vi "Periodic Tasks.vi"(8 "error in":errorcluster) -> ()   [LabVIEW 2019]
doc: "This VI runs in parallel to other tasks. It can contain as many user-defined periodic loops as you need. These can carry out PID or other sorts of timed response."
uses:
  <vilib>/Rock Robotics/WPI/Solenoid/WPI_SolenoidValue.ctl
  <vilib>/Rock Robotics/WPI/Utilities/WPI_GetSetVariantRefNum.vi
  <vilib>/Rock Robotics/Network Tables/NT Write Boolean.vi
  <vilib>/Rock Robotics/WPI/Solenoid/WPI_SolenoidSetEnum.vi
panel:
  in  "Output 3":dbl=-0.8 format="%#_13g"
  in  "Bottom":dbl=-1.0 format="%#_13g"
  in  "Top":dbl=0.27 format="%#_13g"
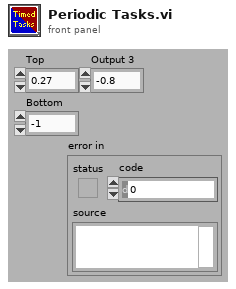
[diagram p1: front panel]
types:
  T1 = typedef "WPI_JoystickDevRef.ctl" = cluster{"Device":T2}
  T2 = typedef "WPI_JoystickDeviceEnum.ctl" = enum16{"USB 0", "USB 1", "USB 2", "USB 3", "USB 4", "USB 5"}
  T3 = typedef "WPI_SolenoidValue.ctl" = enum16{"Off", "On", "Forward", "Reverse"}
  T4 = typedef "WPI_SolenoidDevRef.ctl" = cluster{"DevStatus":errorcluster, "Pneumatics Control Module":u8, "Forward Solenoid Channel":T5, "Reverse Solenoid Channel":T5}
  T5 = typedef "WPI_SolenoidChannel.ctl" = enum8{"Solenoid 0", "Solenoid 1", "Solenoid 2", "Solenoid 3", "Solenoid 4", "Solenoid 5", "Solenoid 6", "Solenoid 7", "Invalid"}
  T6 = typedef "WPI_MotorControlDeviceRef.ctl" = cluster{"DeviceStatus":errorcluster, "Type":T7, "PWM":cluster{"PWM Channel":T8, "DeadBand":T9}, "CAN":cluster{"Device Number":u8, "SetOutput VI Ref":variant, "GetOutput VI Ref":variant, "Enable VI Ref":variant, "Disable VI Ref":variant, "Data":variant}, "Invert":bool, "DIO PWM":cluster{"PWM \"Enable\" Channel":T8, "DIOChannel":T10, "PWM Rate":dbl}}
  T7 = typedef "WPI_MotorControlType.ctl" = enum16{"PWM", "CAN", "DIO PWM"}
  T8 = typedef "FPGA_DIOPWMChannel.ctl" = enum8{"PWM 0", "PWM 1", "PWM 2", "PWM 3", "PWM 4", "PWM 5", "PWM 6", "PWM 7", "PWM 8", "PWM 9", "PWM MXP 0", "PWM MXP 1", "PWM MXP 2", "PWM MXP 3", "PWM MXP 4", "PWM MXP 5", "PWM MXP 6", "PWM MXP 7", "PWM MXP 8", "PWM MXP 9", "Invalid"}
  T9 = typedef "WPI_PWMDeadband.ctl" = cluster{"Name":string, "maxPositivePwm":i32, "minPositivePwm":i32, "centerPwm":i32, "maxNegativePwm":i32, "minNegativePwm":i32, "angularRange":u16}
  T10 = typedef "FPGA_DIOChannel.ctl" = enum8{"DIO 0", "DIO 1", "DIO 2", "DIO 3", "DIO 4", "DIO 5", "DIO 6", "DIO 7", "DIO 8", "DIO 9", "DIO MXP 0", "DIO MXP 1", "DIO MXP 2", "DIO MXP 3", "DIO MXP 4", "DIO MXP 5", "DIO MXP 6", "DIO MXP 7", "DIO MXP 8", "DIO MXP 9", "DIO MXP 10", "DIO MXP 11", "DIO MXP 12", "DIO MXP 13", "DIO MXP 14", "DIO MXP 15", "SPI Port CS1", "SPI Port CS2", "SPI Port CS3", "SPI Port MISO", "SPI Port MOSI", "Invalid"}
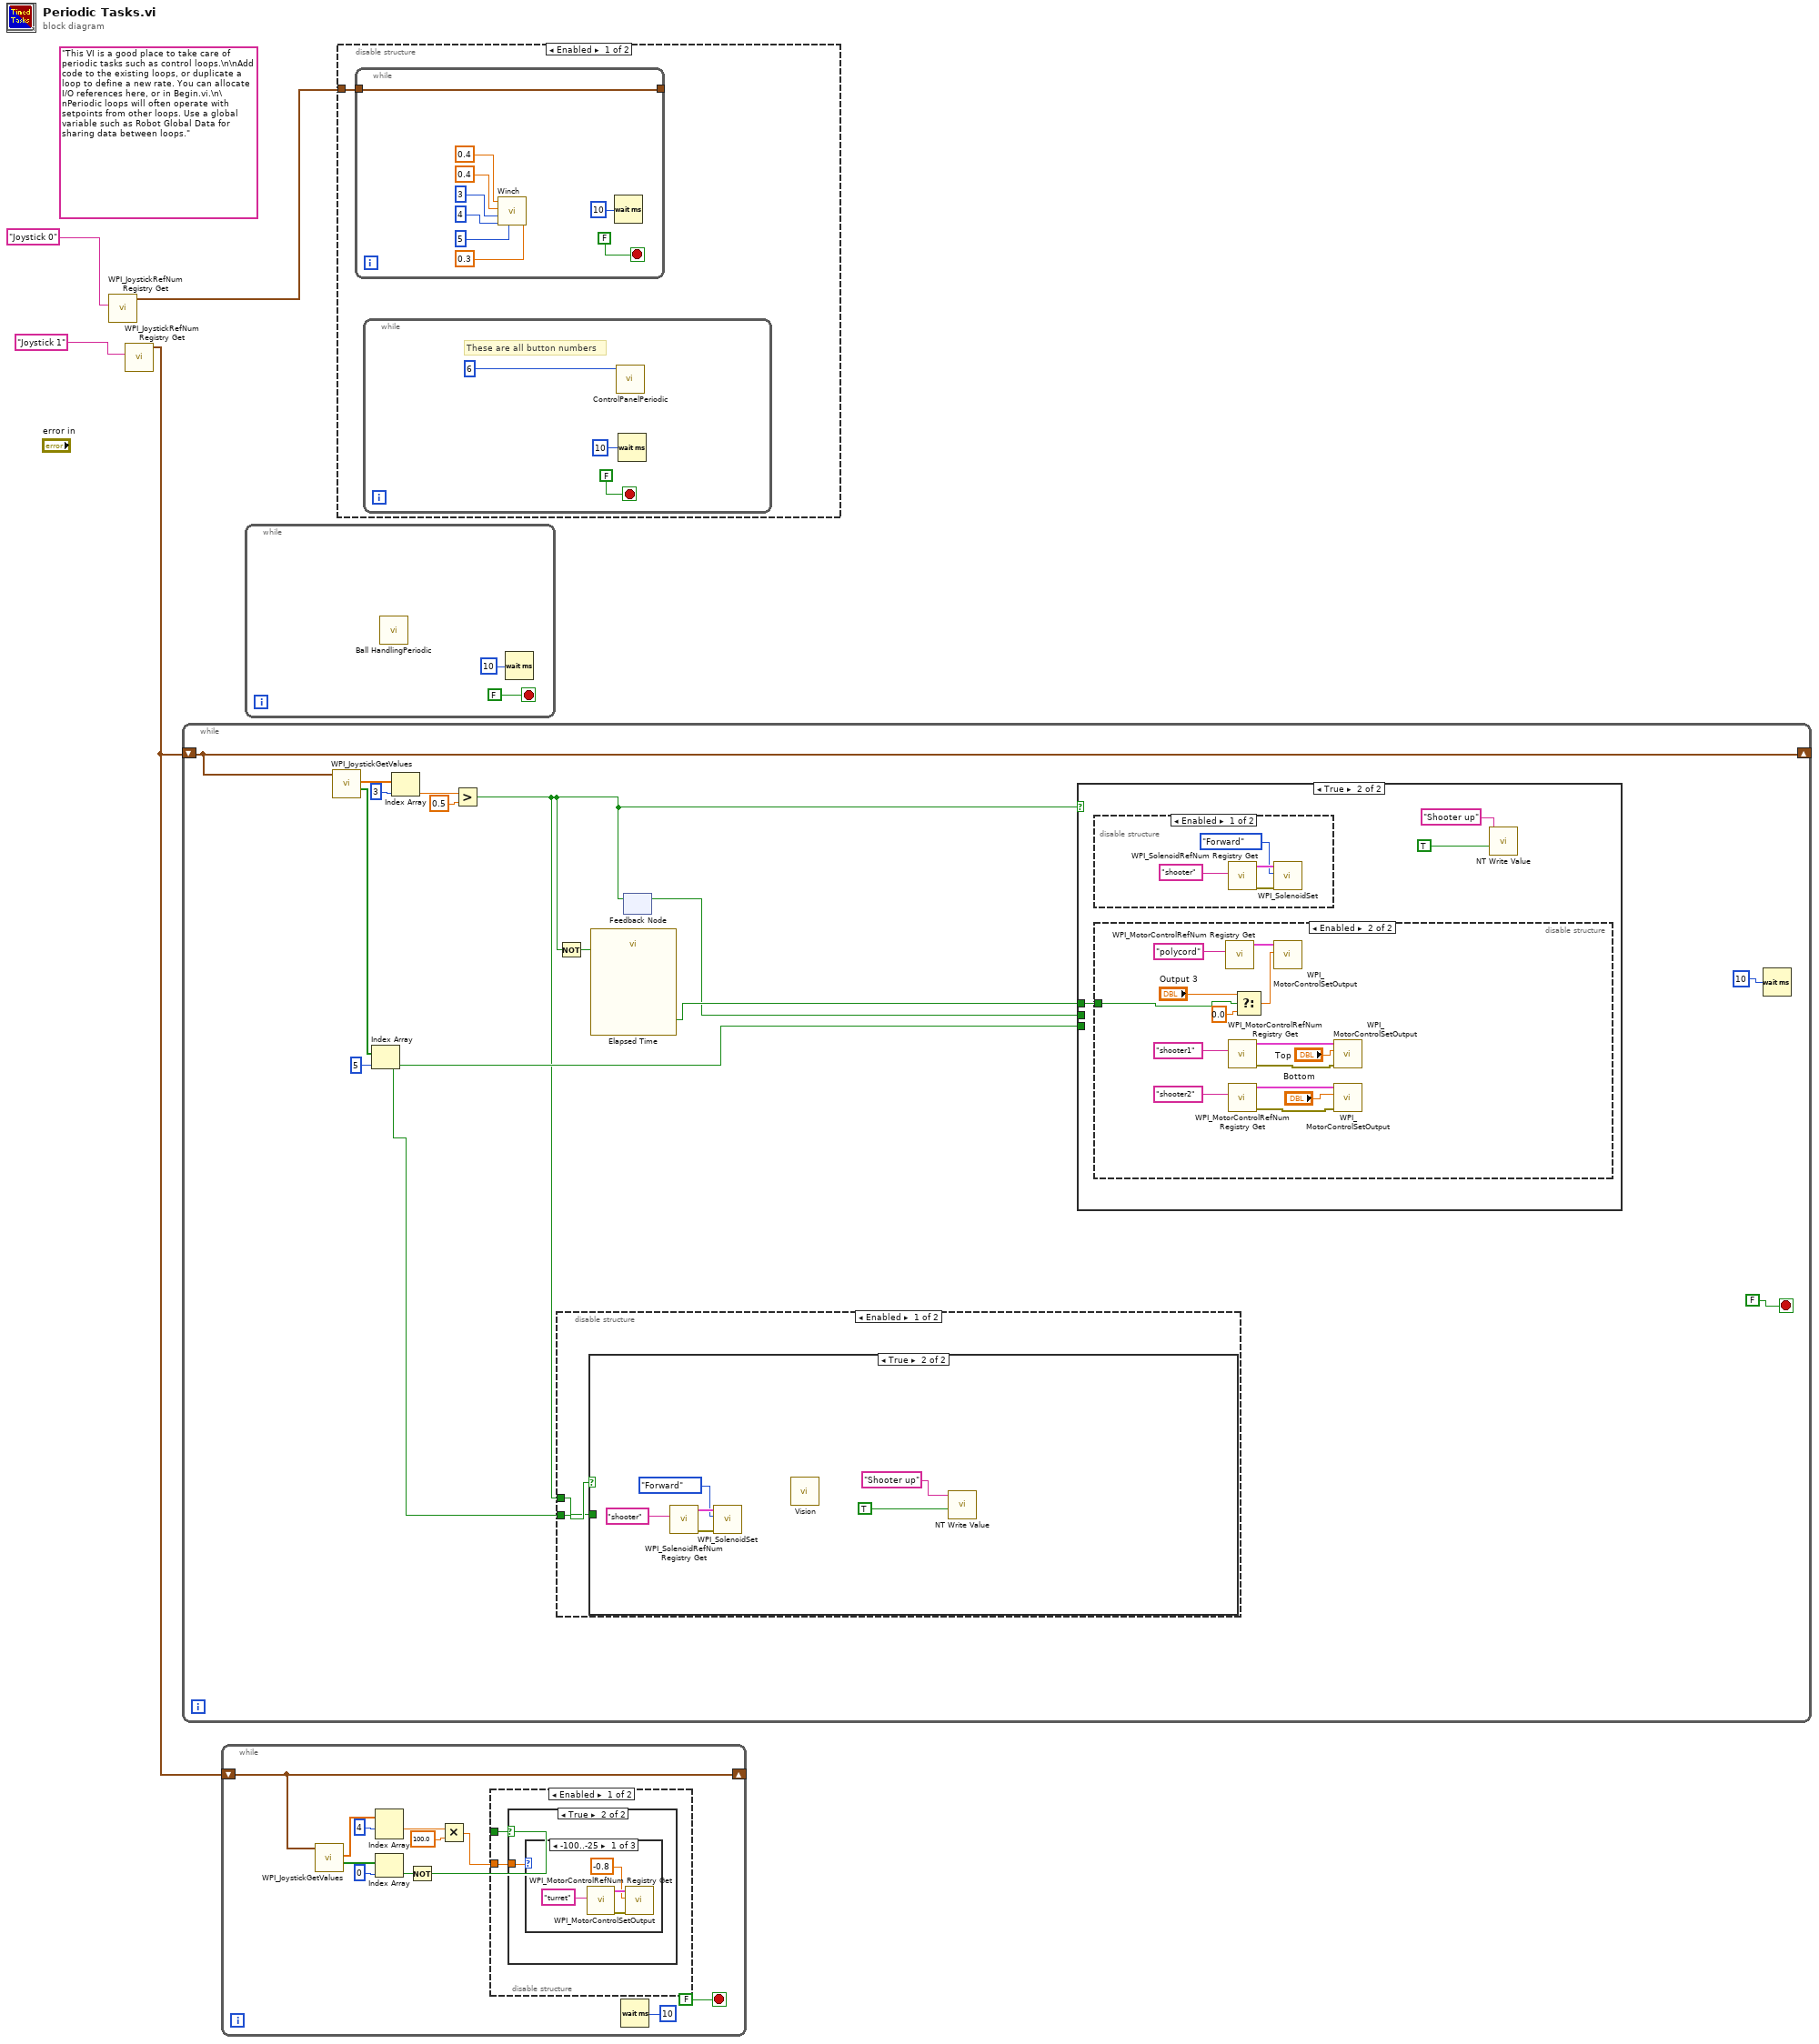
[diagram p0: block diagram]
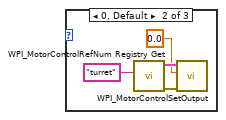
[diagram p3: hidden frame]
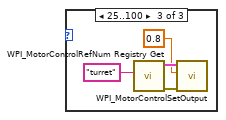
[diagram p4: hidden frame]
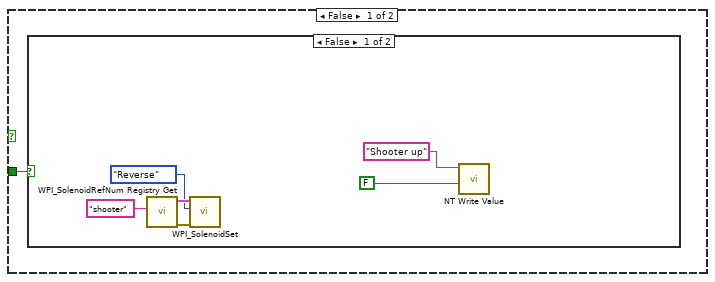
[diagram p6: hidden frame]
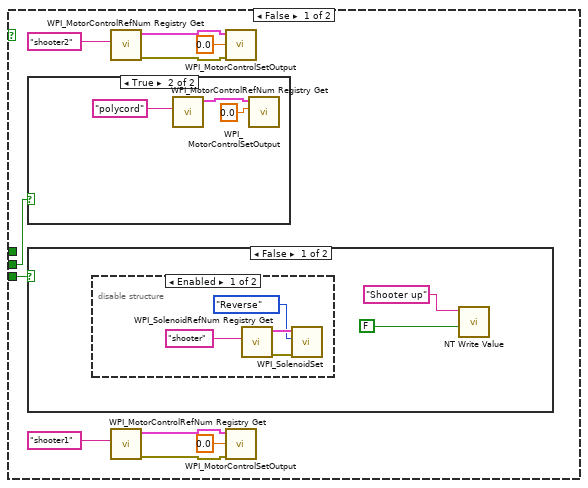
[diagram p9: hidden frame]
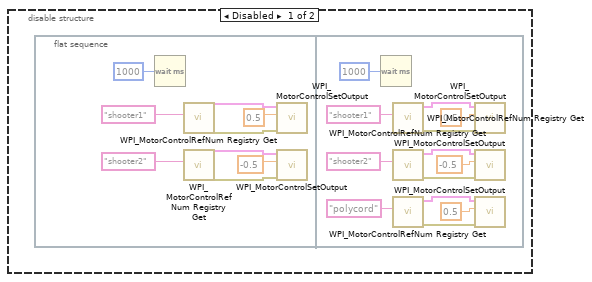
[diagram p14: hidden frame]
diagram:
  (unwired) "This VI is a good place to take care of periodic tasks such as control loops.\n\nAdd code to the existing loops, or duplicate a loop to define a new rate. You can allocate I/O references here, or in Begin.vi.\n\nPeriodic loops will often operate with setpoints from other loops. Use a global variable such as Robot Global Data for sharing data between loops."
  n1 = call <vilib>:"WPI_JoystickRefNum Registry Get.vi"("refnum name"="Joystick 0") -> ("JoystickDevRef"=w3:T1)  [unwired: 1 in, 9 out]
  n2 = call <vilib>:"WPI_JoystickRefNum Registry Get.vi"("refnum name"="Joystick 1") -> ("JoystickDevRef"=w1:T1)  [unwired: 1 in, 9 out]
  n3 = while {
    shift-right: [w16] -> _
    shift-left: w1 -> [w16]
    stop <- FALSE stop-if-true
    n4 = call <vilib>:"WPI_JoystickGetValues.vi"("JoystickDevRef"=w16) -> ("Buttons"=w9:bool[], "Axes"=w15:dbl[])  [unwired: 6 in, 3 out]
    n5 = Index Array(array=w9, index=5) -> (element=w7:bool)
    n6 = Index Array(array=w15, index=3) -> (element=w13:dbl)
    n7 = Greater?(x=w13, y=0.5) -> (0:w6:bool)
    n8 = Not(x=w6) -> (.not. x?=w11:bool)
    n9 = disable-structure shown="Enabled" {
      disable-tunnel: w7 -> [w20 _]
      disable-tunnel: w6 -> [w19 _]
      frame Enabled {
        n10 = case shown="True" w20 {
          tunnel: w19 -> [w21 _]
          frame False {
            n11 = case shown="False" w21 {
              frame False {
                n12 = call <vilib>:"WPI_SolenoidRefNum Registry Get.vi"("refnum name"="shooter") -> ("error out"=w27:errorcluster, "SolenoidDevRef"=w26:T4)  [unwired: 9 in]
                n13 = call-poly <vilib>:"WPI_SolenoidSet.vi"("error in (no error)"=w27, "Value"=WPI_SolenoidValue."Reverse", "SolenoidDevRef"=w26) -> ()  [unwired: 7 in, 2 out]
                n14 = call-poly <vilib>:"NT Write Value.vi"("Boolean"=FALSE, "Name"="Shooter up") -> ()  [unwired: 9 in, 1 out]
              }
              frame True {
              }
            }
          }
          frame True {
            n15 = call <vilib>:"WPI_SolenoidRefNum Registry Get.vi"("refnum name"="shooter") -> ("error out"=w33:errorcluster, "SolenoidDevRef"=w32:T4)  [unwired: 9 in]
            n16 = call-poly <vilib>:"WPI_SolenoidSet.vi"("error in (no error)"=w33, "Value"=WPI_SolenoidValue."Forward", "SolenoidDevRef"=w32) -> ()  [unwired: 7 in, 2 out]
            n17 = call "Vision.vi"() -> ()  [unwired: 12 in]
            n18 = call-poly <vilib>:"NT Write Value.vi"("Boolean"=TRUE, "Name"="Shooter up") -> ()  [unwired: 9 in, 1 out]
          }
        }
      }
      frame Disabled {
      }
    }
    n19 = call "Elapsed Time"("Reset"=w11) -> ("Time has Elapsed"=w10:bool)  [unwired: 11 in, 7 out]
    n20 = feedback-in #1(w6) -> ()
    n21 = feedback #1() -> (w5:bool)  [unwired: 1 in]
    n22 = case shown="True" w6 {
      tunnel: w10 -> [_ w55]
      tunnel: w7 -> [w35 _]
      tunnel: w5 -> [w34 _]
      frame False {
        n23 = case shown="True" w34 {
          frame False {
          }
          frame True {
            n24 = call <vilib>:"WPI_MotorControlRefNum Registry Get.vi"("refnum name"="polycord") -> ("MotorControlDevRef"=w45:T6)  [unwired: 9 in, 1 out]
            n25 = call <vilib>:"WPI_MotorControlSetOutput.vi"("Output"=0.0, "MotorControlDevRef"=w45) -> ()  [unwired: 7 in, 3 out]
          }
        }
        n26 = case shown="False" w35 {
          frame False {
            n27 = disable-structure shown="Enabled" {
              frame Enabled {
                n28 = call <vilib>:"WPI_SolenoidRefNum Registry Get.vi"("refnum name"="shooter") -> ("error out"=w51:errorcluster, "SolenoidDevRef"=w52:T4)  [unwired: 9 in]
                n29 = call-poly <vilib>:"WPI_SolenoidSet.vi"("error in (no error)"=w51, "Value"=WPI_SolenoidValue."Reverse", "SolenoidDevRef"=w52) -> ()  [unwired: 7 in, 2 out]
              }
              frame Disabled {
              }
            }
            n30 = call-poly <vilib>:"NT Write Value.vi"("Boolean"=FALSE, "Name"="Shooter up") -> ()  [unwired: 9 in, 1 out]
          }
          frame True {
          }
        }
        n31 = call <vilib>:"WPI_MotorControlRefNum Registry Get.vi"("refnum name"="shooter2") -> ("error out"=w38:errorcluster, "MotorControlDevRef"=w37:T6)  [unwired: 9 in]
        n32 = call <vilib>:"WPI_MotorControlRefNum Registry Get.vi"("refnum name"="shooter1") -> ("error out"=w42:errorcluster, "MotorControlDevRef"=w41:T6)  [unwired: 9 in]
        n33 = call <vilib>:"WPI_MotorControlSetOutput.vi"("error in (no error)"=w38, "Output"=0.0, "MotorControlDevRef"=w37) -> ()  [unwired: 6 in, 3 out]
        n34 = call <vilib>:"WPI_MotorControlSetOutput.vi"("error in (no error)"=w42, "Output"=0.0, "MotorControlDevRef"=w41) -> ()  [unwired: 6 in, 3 out]
      }
      frame True {
        n35 = disable-structure shown="Enabled" {
          frame Enabled {
            n36 = call <vilib>:"WPI_SolenoidRefNum Registry Get.vi"("refnum name"="shooter") -> ("error out"=w59:errorcluster, "SolenoidDevRef"=w58:T4)  [unwired: 9 in]
            n37 = call-poly <vilib>:"WPI_SolenoidSet.vi"("error in (no error)"=w59, "Value"=WPI_SolenoidValue."Forward", "SolenoidDevRef"=w58) -> ()  [unwired: 7 in, 2 out]
          }
          frame Disabled {
          }
        }
        n38 = disable-structure shown="Enabled" {
          disable-tunnel: w55 -> [_ w85]
          frame Disabled {
            n39 = flat-sequence {
              frame #0 {
                n40 = Wait (ms)(milliseconds to wait=u32 1000) -> ()  [unwired: 1 out]
                n41 = call <vilib>:"WPI_MotorControlRefNum Registry Get.vi"("refnum name"="shooter1") -> ("error out"=w67:errorcluster, "MotorControlDevRef"=w66:T6)  [unwired: 9 in]
                n42 = call <vilib>:"WPI_MotorControlRefNum Registry Get.vi"("refnum name"="shooter2") -> ("error out"=w64:errorcluster, "MotorControlDevRef"=w63:T6)  [unwired: 9 in]
                n43 = call <vilib>:"WPI_MotorControlSetOutput.vi"("error in (no error)"=w67, "Output"=0.5, "MotorControlDevRef"=w66) -> ()  [unwired: 6 in, 3 out]
                n44 = call <vilib>:"WPI_MotorControlSetOutput.vi"("error in (no error)"=w64, "Output"=-0.5, "MotorControlDevRef"=w63) -> ()  [unwired: 6 in, 3 out]
              }
              frame #1 {
                n45 = Wait (ms)(milliseconds to wait=u32 1000) -> ()  [unwired: 1 out]
                n46 = call <vilib>:"WPI_MotorControlRefNum Registry Get.vi"("refnum name"="shooter1") -> ("error out"=w80:errorcluster, "MotorControlDevRef"=w79:T6)  [unwired: 9 in]
                n47 = call <vilib>:"WPI_MotorControlRefNum Registry Get.vi"("refnum name"="shooter2") -> ("error out"=w76:errorcluster, "MotorControlDevRef"=w75:T6)  [unwired: 9 in]
                n48 = call <vilib>:"WPI_MotorControlRefNum Registry Get.vi"("refnum name"="polycord") -> ("error out"=w72:errorcluster, "MotorControlDevRef"=w71:T6)  [unwired: 9 in]
                n49 = call <vilib>:"WPI_MotorControlSetOutput.vi"("error in (no error)"=w80, "Output"=0.5, "MotorControlDevRef"=w79) -> ()  [unwired: 6 in, 3 out]
                n50 = call <vilib>:"WPI_MotorControlSetOutput.vi"("error in (no error)"=w76, "Output"=-0.5, "MotorControlDevRef"=w75) -> ()  [unwired: 6 in, 3 out]
                n51 = call <vilib>:"WPI_MotorControlSetOutput.vi"("error in (no error)"=w72, "Output"=0.5, "MotorControlDevRef"=w71) -> ()  [unwired: 6 in, 3 out]
              }
            }
          }
          frame Enabled {
            n52 = call <vilib>:"WPI_MotorControlRefNum Registry Get.vi"("refnum name"="polycord") -> ("MotorControlDevRef"=w86:T6)  [unwired: 9 in, 1 out]
            n53 = call <vilib>:"WPI_MotorControlRefNum Registry Get.vi"("refnum name"="shooter1") -> ("error out"=w94:errorcluster, "MotorControlDevRef"=w93:T6)  [unwired: 9 in]
            n54 = call <vilib>:"WPI_MotorControlRefNum Registry Get.vi"("refnum name"="shooter2") -> ("error out"=w90:errorcluster, "MotorControlDevRef"=w89:T6)  [unwired: 9 in]
            n55 = Select(t="Output 3", s=w85, f=0.0) -> (s? t:f=w83:dbl)
            n56 = call <vilib>:"WPI_MotorControlSetOutput.vi"("Output"=w83, "MotorControlDevRef"=w86) -> ()  [unwired: 7 in, 3 out]
            n57 = call <vilib>:"WPI_MotorControlSetOutput.vi"("error in (no error)"=w94, "Output"="Top", "MotorControlDevRef"=w93) -> ()  [unwired: 6 in, 3 out]
            n58 = call <vilib>:"WPI_MotorControlSetOutput.vi"("error in (no error)"=w90, "Output"="Bottom", "MotorControlDevRef"=w89) -> ()  [unwired: 6 in, 3 out]
          }
        }
        n59 = call-poly <vilib>:"NT Write Value.vi"("Boolean"=TRUE, "Name"="Shooter up") -> ()  [unwired: 9 in, 1 out]
      }
    }
    n60 = Wait (ms)(milliseconds to wait=u32 10) -> ()  [unwired: 1 out]
  }
  n61 = while {
    shift-right: [w105] -> _
    shift-left: w1 -> [w105]
    stop <- FALSE stop-if-true
    n62 = call <vilib>:"WPI_JoystickGetValues.vi"("JoystickDevRef"=w105) -> ("Buttons"=w98:bool[], "Axes"=w104:dbl[])  [unwired: 6 in, 3 out]
    n63 = Index Array(array=w104, index #1=4 ("index")) -> (element #1=w102:dbl)  [unwired: 1 in, 1 out]
    n64 = Index Array(array=w98, index=0) -> (element=w97:bool)
    n65 = Not(x=w97) -> (.not. x?=w96:bool)
    n66 = Multiply(x=w102, y=100.0) -> (x*y=w100:dbl)
    n67 = disable-structure shown="Enabled" {
      disable-tunnel: w100 -> [w109 _]
      disable-tunnel: w96 -> [w108 _]
      frame Enabled {
        n68 = case shown="True" w108 {
          tunnel: w109 -> [_ w110]
          frame False {
          }
          frame True {
            n69 = case shown="-100..-25" w110 {
              frame -100..-25 {
                n70 = call <vilib>:"WPI_MotorControlRefNum Registry Get.vi"("refnum name"="turret") -> ("error out"=w113:errorcluster, "MotorControlDevRef"=w112:T6)  [unwired: 9 in]
                n71 = call <vilib>:"WPI_MotorControlSetOutput.vi"("error in (no error)"=w113, "Output"=-0.8, "MotorControlDevRef"=w112) -> ()  [unwired: 6 in, 3 out]
              }
              frame 0, Default {
                n72 = call <vilib>:"WPI_MotorControlRefNum Registry Get.vi"("refnum name"="turret") -> ("error out"=w117:errorcluster, "MotorControlDevRef"=w116:T6)  [unwired: 9 in]
                n73 = call <vilib>:"WPI_MotorControlSetOutput.vi"("error in (no error)"=w117, "Output"=0.0, "MotorControlDevRef"=w116) -> ()  [unwired: 6 in, 3 out]
              }
              frame 25..100 {
                n74 = call <vilib>:"WPI_MotorControlRefNum Registry Get.vi"("refnum name"="turret") -> ("error out"=w121:errorcluster, "MotorControlDevRef"=w120:T6)  [unwired: 9 in]
                n75 = call <vilib>:"WPI_MotorControlSetOutput.vi"("error in (no error)"=w121, "Output"=0.8, "MotorControlDevRef"=w120) -> ()  [unwired: 6 in, 3 out]
              }
            }
          }
        }
      }
      frame Disabled {
      }
    }
    n76 = Wait (ms)(milliseconds to wait=u32 10) -> ()  [unwired: 1 out]
  }
  n77 = while {
    stop <- FALSE stop-if-true
    n78 = call "Ball HandlingPeriodic.vi"() -> ()  [unwired: 12 in]
    n79 = Wait (ms)(milliseconds to wait=u32 10) -> ()  [unwired: 1 out]
  }
  n80 = disable-structure shown="Enabled" {
    disable-tunnel: w3 -> [w125 _]
    frame Enabled {
      n81 = while {
        tunnel: w125 -> [w135]
        tunnel: [w135] -> _
        stop <- FALSE stop-if-true
        n82 = call "Winch.vi"("Color Elevator speed"=0.3, "ElevatorButtonDown"=5, "WinchButton"=4 ("button"), "ElevatorButtonUp"=3 ("ElevatorButton"), "WinchSpeed"=0.4 ("Speed"), "ElevatorSpeed"=0.4) -> ()  [unwired: 6 in]
        n83 = Wait (ms)(milliseconds to wait=u32 10) -> ()  [unwired: 1 out]
      }
      n84 = while {
        stop <- FALSE stop-if-true
        # "These are all button numbers"
        n85 = call "ControlPanelPeriodic.vi"("One color"=6) -> ()  [unwired: 11 in]
        n86 = Wait (ms)(milliseconds to wait=u32 10) -> ()  [unwired: 1 out]
      }
    }
    frame Disabled {
    }
  }
